vi "USRP Config.vi"(0 "USRP Configuration":T1={"USRP RIO Resources"=["USRP-2945"], "LO Sharing"=TRUE, "Carrier Frequency (Hz)"=2000000000.0, "Gain"=40.0, "Sample rate (Hz)"=100000000.0, "reference frequency source"="Internal", "start trigger"=enum."Software"} {"Sample rate (Hz)" format="%#_6p"; "Carrier Frequency (Hz)" format="%#_6p"}, 2 "Simulate and check Data":bool, 11 "error in (no error)":errorcluster) -> (4 "Array":T4[](array[typedef]) {"Daughterboard Clock Rate" format="%#.3pHz"; "FPGA Data Clock Rate" format="%#.3pHz"; "Data Clock Rate" format="%#.3pHz"; "Characterization Data"."Frequencies [Hz]" format="%#_6p"; "EEPROM Characterization Header"."Pointer to Device Data Header" format="%x"; "EEPROM Characterization Header"."Checksum" format="%x"; "Device Data Header"."Pointer to Characterization Data" format="%x"; "Device Data Header"."Checksum" format="%x"; "EEPROM Header"."Pointer to User Header" format="%x"; "EEPROM Header"."Pointer to Factory Header" format="%x"; "EEPROM Header"."Product Code" format="%x"; "EEPROM Header"."Checksum" format="%x"}, 6 "start trigger out":T3, 8 "USRP RIO Ports":bool[](array[boolean])=[TRUE, TRUE], 10 "Time Stamp":timestamp, 14 "rx.enabled channels":string[][](array[string]), 15 "error out":errorcluster)   [LabVIEW 2016]
uses:
  <instrlib>/niUsrpRio/Config/v1/Host/Public/niUsrpRio Session.ctl
  <instrlib>/_niInstr/Register Bus/v0/Host/Public/Register Bus Session.ctl
  <instrlib>/_niInstr/Register Bus/v0/Host/Private/Session Data.ctl
  <instrlib>/niUsrpRio/Config/v1/Host/Private/DB Queue Reference.ctl
  <instrlib>/niUsrpRio/Config/v1/Host/Private/Daughterboard Data.ctl
  <instrlib>/niUsrpRio/Config/v1/Host/Private/ATR state data.ctl
  <instrlib>/niUsrpRio/Config/v1/Host/Private/Antenna Configuration.ctl
  <instrlib>/niUsrpRio/Config/v1/Host/Private/CPLD Power Mode.ctl
  <instrlib>/niUsrpRio/Config/v1/Host/Public/EEPROM Header.ctl
  <instrlib>/niUsrpRio/Config/v1/Host/Public/EEPROM Device Data Header.ctl
  <instrlib>/niUsrpRio/Config/v1/Host/Public/EEPROM Characterization Header.ctl
  <instrlib>/niUsrpRio/Config/v1/Host/Public/Characterization Data.ctl
  <instrlib>/niUsrpRio/Config/v1/Host/Public/IQ Imbalance.ctl
  29x5/SubVIs/Start Trigger.ctl
  TypeDefs/USRP Configuration.ctl
  <vilib>/userdefined/Silver/nirio_resource_slv.ctl
  <instrlib>/_niInstr/Register Bus/v0/Host/niInstr Register Bus v0 Host.lvlib
  <instrlib>/niUsrpRio/Config/v1/Host/niUsrpRio Config v1 Host.lvlib
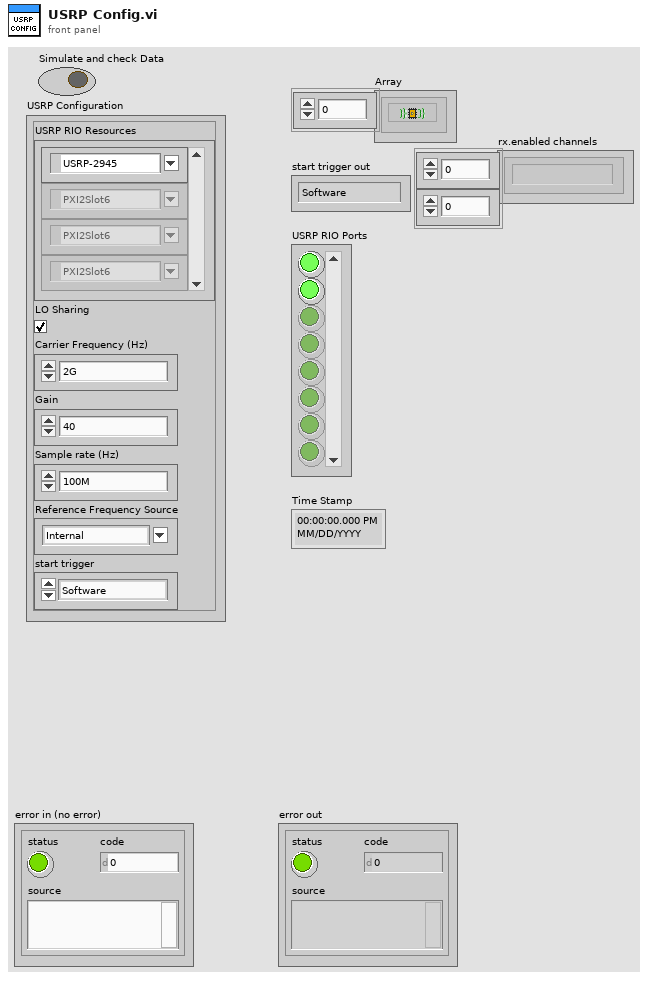
[diagram p1: front panel]
types:
  T1 = typedef "USRP Configuration.ctl" = cluster{"USRP RIO Resources":T2[], "LO Sharing":bool, "Carrier Frequency (Hz)":dbl, "Gain":dbl, "Sample rate (Hz)":dbl, "reference frequency source":string, "start trigger":T3}
  T2 = typedef "nirio_resource_slv.ctl" = tag
  T3 = typedef "Start Trigger.ctl" = enum8{"Software", "Digital Edge", "Rx Start Trigger", "Tx Start Trigger", "Immediate", "Future Time Event"}
  T4 = typedef "niUsrpRio Config v1 Host.lvlib/niUsrpRio Session.ctl" = cluster{"FPGA Interface":refnum<k20>, "RIO Interface Number":u32, "Data Clock Rate":u32, "FPGA Data Clock Rate":u32, "Global Settings Register Bus":T5, "Radio 0 Settings Register Bus":T5, "Radio 1 Settings Register Bus":T5, "Radio Settings Bus Semaphore":T6, "DB Queues":T7[], "Characterization Data Valid?":bool, "EEPROM Header":T8, "Device Data Header":T9, "EEPROM Characterization Header":T10, "Characterization Data":T11[], "FPGA Current Version":u32, "FPGA Oldest Compatible Version":u32, "Fixed Logic Current Version":u32, "Fixed Logic Oldest Compatible Version":u32, "FPGA Radio Settings Bus Current Version":u32, "FPGA Radio Settings Bus Oldest Compatible Version":u32, "FPGA Board Config Current Version":u32, "FPGA Board Config Oldest Compatible Version":u32, "Daughterboard Clock Rate":u32, "daughterboard configuration session handles":u64[]}
  T5 = typedef "niInstr Register Bus v0 Host.lvlib/Register Bus Session.ctl" = refnum<queue>
  T6 = typedef "Semaphore RefNum" = refnum<k1>
  T7 = typedef "niUsrpRio Config v1 Host.lvlib/DB Queue Reference.ctl" = refnum<queue>
  T8 = typedef "niUsrpRio Config v1 Host.lvlib/EEPROM Header.ctl" = cluster{"Checksum":u32, "Product Code":u16, "Hardware Current Version":u16, "Hardware Oldest Compatible Version":u16, "EEPROM Map Current Version":u16, "EEPROM Map Oldest Compatible Version":u16, "User Password":string, "Pointer to Factory Header":u32, "Pointer to User Header":u32, "Recommended Interval":u16, "Number of Reserved Bytes":i32, "Number of Daughterboards":u8, "Daughterboard IDs":u16[], "Daughterboard Serial Numbers":string[]}
  T9 = typedef "niUsrpRio Config v1 Host.lvlib/EEPROM Device Data Header.ctl" = cluster{"Checksum":u32, "Number of Channels":u8, "Number of Gain Settings":u16[], "Pointer to Characterization Data":u32[], "Number of Reserved Bytes":i32, "Number of Frequencies":u16[]}
  T10 = typedef "niUsrpRio Config v1 Host.lvlib/EEPROM Characterization Header.ctl" = cluster{"Checksum":u32, "Date":timestamp, "Temperature":sgl, "Misc. Info":string, "Pointer to Device Data Header":u32, "Number of Reserved Bytes":i32}
  T11 = typedef "niUsrpRio Config v1 Host.lvlib/Characterization Data.ctl" = cluster{"Gains[dB]":dbl[], "Frequencies [Hz]":dbl[], "IQ Imbalance Table":T12[], "Measured Gains[dB]":dbl[][]}
  T12 = typedef "niUsrpRio Config v1 Host.lvlib/IQ Imbalance.ctl" = cluster{"Gain Imbalance [linear]":dbl, "Phase Imbalance [radians]":dbl, "Offset":cdb}
  T13 = enum16{"Independent", "Import", "Shared and Export"}
  T14 = cluster{"transfer mode":enum16{"Finite", "Continuous"}, "sample rate":dbl, "number of samples":u32, "start trigger":T3, "daughterboard 0 config":cluster{"rf enable 0":bool, "rf config 0":cluster{"antenna":string, "frequency":dbl, "gain":dbl}, "rf enable 1":bool, "rf config 1":cluster{"antenna":string, "frequency":dbl, "gain":dbl}, "lo configuration":enum16{"Independent", "Import"}}, "daughterboard 1 config":cluster{"rf enable 2":bool, "rf config 2":cluster{"antenna":string, "frequency":dbl, "gain":dbl}, "rf enable 3":bool, "rf config 3":cluster{"antenna":string, "frequency":dbl, "gain":dbl}, "lo configuration":enum16{"Independent", "Import", "Shared and Export"}}}
  T15 = typedef "Rx Channels.ctl" = cluster{"rx config":cluster{"channel configuration":cluster{"channel enable":bool, "channel configuration":cluster{"antenna":string, "frequency":dbl, "lo frequency":dbl, "level":dbl}}[], "transfer mode":enum16{"Finite", "Continuous"}, "sample rate":dbl, "number of samples":u32, "start trigger":T3}, "reference frequency source":string, "rx.data sink":enum16{"SFP Port 0", "SFP Port 1", "Host"}, "rx.enabled channels":string[], "vertical range":dbl[], "rx.coerced configurations":cluster{"coerced frequencies":dbl[], "coerced lo frequencies":dbl[], "coerced levels":dbl[], "coerced sample rates":dbl[]}}
  T16 = cluster{"coerced frequencies":dbl[], "coerced if1 frequencies":dbl[], "coerced if2 frequencies":dbl[], "coerced gain":dbl[], "coerced sample rates":dbl[]}
  T17 = cluster{"hard error":bool, "soft error":bool, "lane up":bool, "channel up":bool, "sys reset":bool}[]
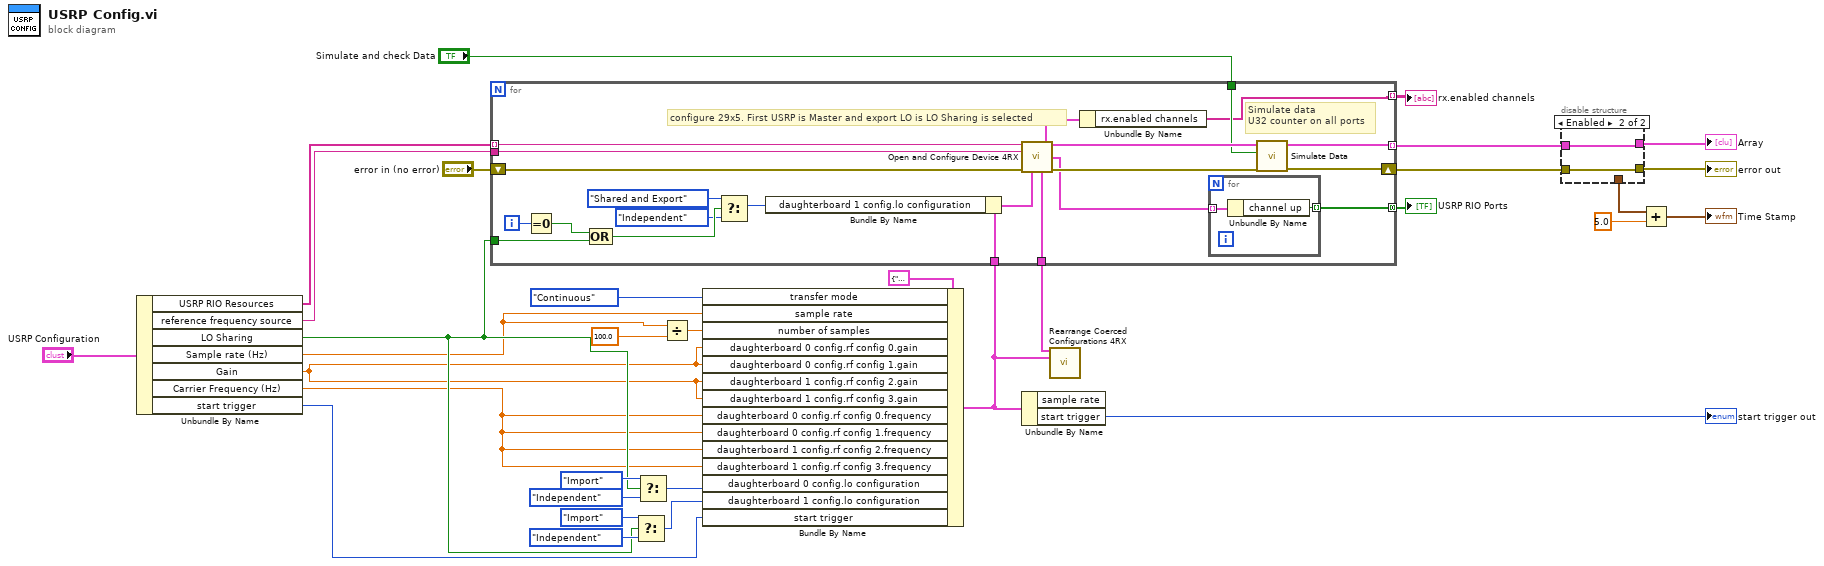
[diagram p0: block diagram]
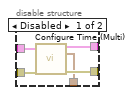
[diagram p2: hidden frame]
diagram:
  n1 = Unbundle By Name("USRP Configuration") -> ("USRP RIO Resources"=w8:T2[], "reference frequency source"=w7:string, "LO Sharing"=w6:bool, "Sample rate (Hz)"=w5:dbl, "Gain"=w4:dbl, "Carrier Frequency (Hz)"=w3:dbl, "start trigger"=w2:T3)
  n2 = Select(t=T13."Import" ("daughterboard 1 config.lo configuration"), s=w6, f=T13."Independent") -> (s? t:f=w24:T13)
  n3 = Select(t=enum16{"Independent", "Import"}."Import" ("daughterboard 0 config.lo configuration"), s=w6, f=enum16{"Independent", "Import"}."Independent") -> (s? t:f=w16:enum16{"Independent", "Import"})
  n4 = Divide(x=w5, y=100.0) -> (x/y=w13:dbl)
  n5 = Bundle By Name(cluster=T14 {"transfer mode"=enum."Finite", "sample rate"=10000000.0, "number of samples"=8192, "start trigger"=enum."Software", "daughterboard 0 config"={"rf enable 0"=TRUE, "rf config 0"={"antenna"="RX1", "frequency"=5000000000.0, "gain"=40.0}, "rf enable 1"=TRUE, "rf config 1"={"antenna"="RX2", "frequency"=5000000000.0, "gain"=40.0}, "lo configuration"=enum."Independent"}, "daughterboard 1 config"={"rf enable 2"=TRUE, "rf config 2"={"antenna"="RX1", "frequency"=5000000000.0, "gain"=40.0}, "rf enable 3"=TRUE, "rf config 3"={"antenna"="RX2", "frequency"=5000000000.0, "gain"=40.0}, "lo configuration"=enum."Independent"}} ("rx config"), "transfer mode"=enum16{"Finite", "Continuous"}."Continuous", "sample rate"=w5, "number of samples"=w13, "daughterboard 0 config.rf config 0.gain"=w4, "daughterboard 0 config.rf config 1.gain"=w4, "daughterboard 1 config.rf config 2.gain"=w4, "daughterboard 1 config.rf config 3.gain"=w4, "daughterboard 0 config.rf config 0.frequency"=w3, "daughterboard 0 config.rf config 1.frequency"=w3, "daughterboard 1 config.rf config 2.frequency"=w3, "daughterboard 1 config.rf config 3.frequency"=w3, "daughterboard 0 config.lo configuration"=w16, "daughterboard 1 config.lo configuration"=w24, "start trigger"=w2) -> (w23:T14)
  n6 = for {
    tunnel: w7 -> [w35]
    tunnel: w8 -> [w54] mode=indexing
    tunnel: [w53] -> w10
    tunnel: w23 -> [w50]
    shift-right: [w40] -> w27
    shift-left: "error in (no error)" -> [w52]
    tunnel: [w39] -> w32 mode=indexing
    tunnel: w6 -> [w45]
    tunnel: "Simulate and check Data" -> [w38]
    tunnel: [w36] -> w26 mode=concatenating
    tunnel: [w33] -> w1 mode=indexing
    i -> [w49]
    # "Simulate data\nU32 counter on all ports"
    # "configure 29x5. First USRP is Master and export LO is LO Sharing is selected"
    n7 = Equal To 0?(x=w49) -> (x = 0?=w46:bool)
    n8 = Compound Arithmetic op=OR(w46, w45) -> (w44:bool)
    n9 = Select(t=T13."Shared and Export" ("daughterboard 1 config.lo configuration"), s=w44, f=T13."Independent") -> (s? t:f=w48:T13)
    n10 = Bundle By Name(cluster=w50, "daughterboard 1 config.lo configuration"=w48) -> (w51:T14)
    n11 = call "Open and Configure Device 4RX.vi"("USRP RIO Device"=w54, "reference frequency source"=w35, "error in"=w52, "rx config"=w51) -> ("rx channels"=w34:T15, "niUsrpRio Session (out)"=w42:T4, "rx.coerced configurations"=w53:T16, "Ports debug"=w37:T17, "error out"=w41:errorcluster)  [unwired: 7 in]
    n12 = Unbundle By Name(w34) -> ("rx.enabled channels"=w33:string[])
    n13 = for {
      tunnel: w37 -> [w56] mode=indexing
      tunnel: [w55] -> w36 mode=indexing
      n14 = Unbundle By Name(w56) -> ("channel up"=w55:bool)
    }
    n15 = call "Simulate Data.vi"("Error In"=w41, "Simulate Data"=w38, "niUsrpRio Session in"=w42) -> ("Error Out"=w40:errorcluster, "niUsrpRio Session out"=w39:T4)  [unwired: 7 in]
  }
  "USRP RIO Ports" <- w26
  "rx.enabled channels" <- w1
  n16 = Unbundle By Name(w23) -> ("start trigger"=→"start trigger out":T3)  [unwired: 1 out]
  n17 = call "Rearrange Coerced Configurations 4RX.vi"("rx.coerced configurations"=w10, "rx config"=w23) -> ()  [unwired: 13 in, 1 out]
  n18 = disable-structure shown="Enabled" {
    disable-tunnel: w32 -> [w61 w63]
    disable-tunnel: w27 -> [w60 w62]
    disable-tunnel: [w59 w62] -> w28
    disable-tunnel: [w58 w63] -> w29
    disable-tunnel: [w57 _] -> w30
    frame Disabled {
      n19 = call "Configure Time (Multi).vi"("niUsrpRio Sessions"=w61, "error in"=w60) -> ("niUsrpRio Sessions (out)"=w58:T4[], "time"=w57:timestamp, "error out"=w59:errorcluster)  [unwired: 11 in]
    }
    frame Enabled {
    }
  }
  "Array" <- w29
  "error out" <- w28
  n20 = Add(x=w30, y=5.0) -> (x+y=→"Time Stamp":timestamp)
